vi "Log Prompt.vi"() -> (3 "prompt":string="Check my datalogger through MCP. Which channels are connected? Identify the channels that have not just noise on them, then log the connected channels for a moment, then stop and read the log file if the log was successful.")   [LabVIEW 2020]
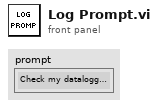
[diagram p1: front panel]
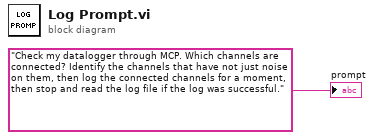
[diagram p0: block diagram]
diagram:
  "prompt" <- "Check my datalogger through MCP. Which channels are connected? Identify the channels that have not just noise on them, then log the connected channels for a moment, then stop and read the log file if the log was successful."
